vi "設定項目_登録_INI書込サブ.vi"(2 "CSV項目名":T1, 4 "設定クラスタ_設定入力":T5 {"測定モード" items=["単発測定モード", "連続測定モード", "多点測定モード"]}, 5 "セレクション(設定)":string, 6 "エラー入力":errorcluster caption="エラー入力 (エラーなし)", 7 "セレクション(No)":string, 8 "使用ON/OFFボタン_設定入力":T3, 9 "キー(配列No)":string[](array[string]), 10 "No設定クラスタ_設定入力":T4, 11 "Refnum入力":T2 caption="refnum") -> (0 "エラー出力":errorcluster, 3 "Refnum出力":T2 caption="refnum")   [LabVIEW 2021]
uses:
  <vilib>/Utility/config.llb/Config Data RefNum.ctl
  <vilib>/Utility/config.llb/Write Key (Double).vi
  <vilib>/Utility/config.llb/Write Key (String).vi
  <vilib>/Utility/config.llb/Write Key (U32).vi
  <vilib>/Utility/config.llb/Write Key (Boolean).vi
  <vilib>/Utility/config.llb/NI_LVConfig.lvlib
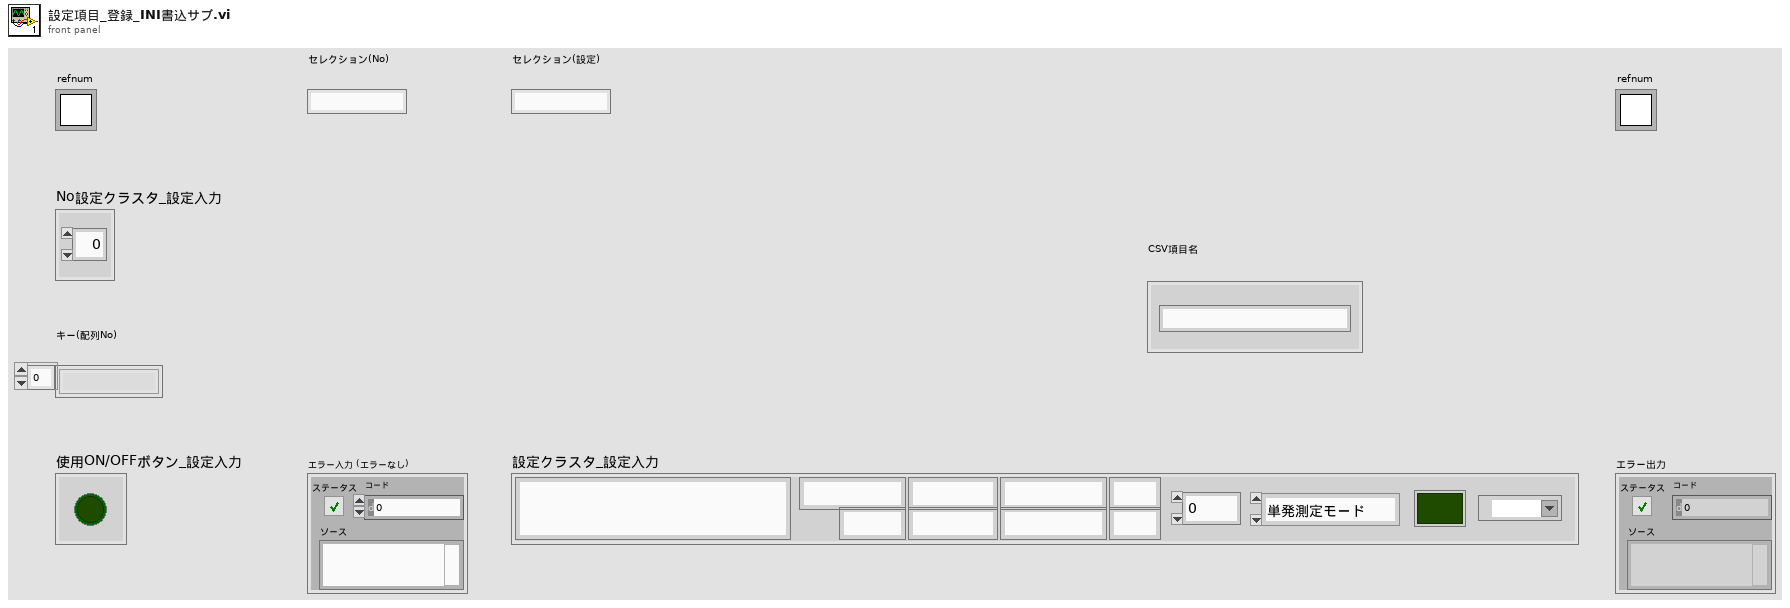
[diagram p1: front panel]
types:
  T1 = typedef "CSV項目名入力.ctl" = cluster{"CSV項目名":string}
  T2 = typedef "NI_LVConfig.lvlib/Config Data RefNum.ctl" = refnum<k1>
  T3 = typedef "ONOFFボタン制御器.ctl" = cluster{"使用ON/OFF":bool}
  T4 = typedef "CH設定表示器.ctl" = cluster{"No. ":dbl}
  T5 = typedef "設定全項目制御器.ctl" = cluster{"規格":string, "規格上限":string, "規格下限":string, "ポートNo.":dbl, "測定モード":u16, "規格単位":string, "品質チェック項目":string, "測定周期":dbl, "実測値MAX":string, "実測値MIN":string, "実測値(MAX)":string, "実測値(MIN)":string, "測定画面表示ボタン":bool, "ゲージポートNo":refnum<visa-resource-name>}
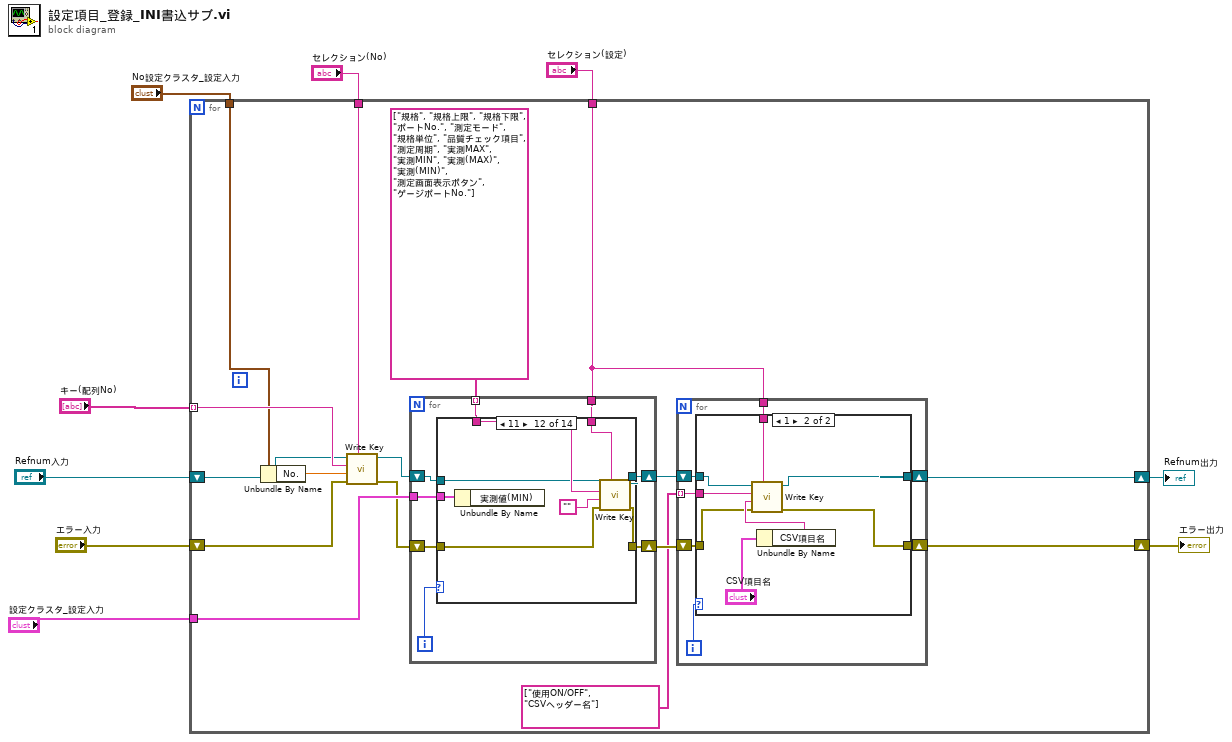
[diagram p0: block diagram]
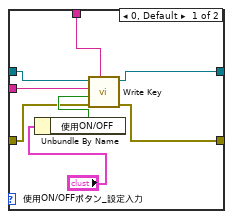
[diagram p2: hidden frame]
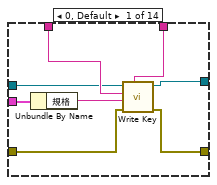
[diagram p3: hidden frame]
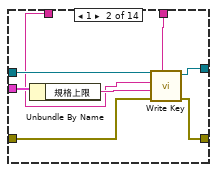
[diagram p4: hidden frame]
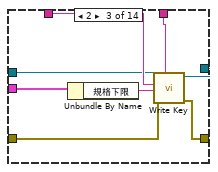
[diagram p5: hidden frame]
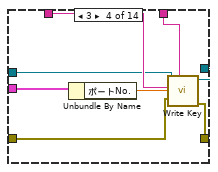
[diagram p6: hidden frame]
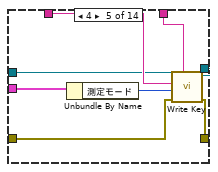
[diagram p7: hidden frame]
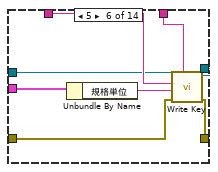
[diagram p8: hidden frame]
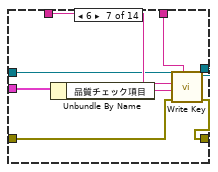
[diagram p9: hidden frame]
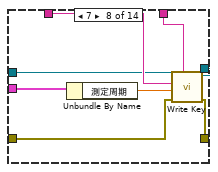
[diagram p10: hidden frame]
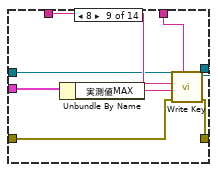
[diagram p11: hidden frame]
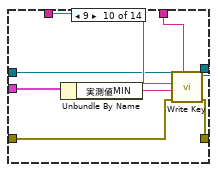
[diagram p12: hidden frame]
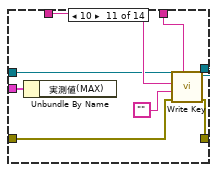
[diagram p13: hidden frame]
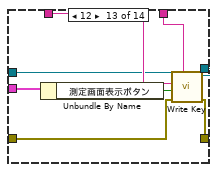
[diagram p14: hidden frame]
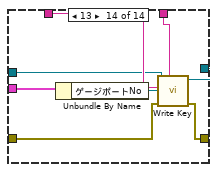
[diagram p15: hidden frame]
diagram:
  n1 = for {
    shift-right: [w23] -> w4
    shift-left: "Refnum入力" -> [w24]
    tunnel: "キー(配列No)" -> [w25] mode=indexing
    shift-right: [w21] -> w5
    shift-left: "エラー入力" -> [w22]
    tunnel: "No設定クラスタ_設定入力" -> [w20]
    tunnel: "設定クラスタ_設定入力" -> [w19]
    tunnel: "セレクション(No)" -> [w18]
    tunnel: "セレクション(設定)" -> [w17]
    n2 = Unbundle By Name(w20) -> ("No."=w16:dbl)
    n3 = call-poly <vilib>:"Write Key.vi"("section"=w18, "error in (no error)"=w22, "value"=w16, "key"=w25, "refnum"=w24) -> ("error out"=w13:errorcluster, "refnum out"=w15:T2)  [unwired: 3 in, 2 out]
    n4 = for {
      shift-right: [w54] -> w14
      shift-left: w15 -> [w56]
      tunnel: string[] ["規格", "規格上限", "規格下限", "ポートNo.", "測定モード", "規格単位", "品質チェック項目", "測定周期", "実測MAX", "実測MIN", "実測(MAX)", "実測(MIN)", "測定画面表示ボタン", "ゲージポートNo."] -> [w55] mode=indexing
      shift-right: [w51] -> w12
      shift-left: w13 -> [w52]
      tunnel: w19 -> [w50]
      tunnel: w17 -> [w49]
      i -> [w53]
      n5 = case shown="11" w53 {
        tunnel: w50 -> [w64 w72 w79 w87 w95 w103 w111 w119 w127 w135 w144 w152 w159 w167]
        tunnel: w55 -> [w62 w69 w78 w86 w94 w102 w110 w118 w126 w134 w143 w151 w158 w166]
        tunnel: w56 -> [w61 w71 w77 w85 w93 w101 w109 w117 w125 w133 w142 w150 w157 w165]
        tunnel: [w60 w67 w76 w84 w92 w100 w108 w116 w124 w132 w141 w149 w156 w164] -> w54
        tunnel: w49 -> [w59 w68 w75 w83 w91 w99 w107 w115 w123 w131 w140 w148 w155 w163]
        tunnel: w52 -> [w58 w66 w74 w82 w90 w98 w106 w114 w122 w130 w139 w147 w154 w162]
        tunnel: [w57 w65 w73 w81 w89 w97 w105 w113 w121 w129 w138 w146 w153 w161] -> w51
        frame 0, Default {
          n6 = Unbundle By Name(w64) -> ("規格"=w63:string)
          n7 = call-poly <vilib>:"Write Key.vi"("section"=w59, "error in (no error)"=w58, "value"=w63, "key"=w62, "refnum"=w61) -> ("error out"=w57:errorcluster, "refnum out"=w60:T2)  [unwired: 1 in, 4 out]
        }
        frame 1 {
          n8 = Unbundle By Name(w72) -> ("規格上限"=w70:string)
          n9 = call-poly <vilib>:"Write Key.vi"("section"=w68, "error in (no error)"=w66, "value"=w70, "key"=w69, "refnum"=w71) -> ("error out"=w65:errorcluster, "refnum out"=w67:T2)  [unwired: 1 in, 4 out]
        }
        frame 2 {
          n10 = Unbundle By Name(w79) -> ("規格下限"=w80:string)
          n11 = call-poly <vilib>:"Write Key.vi"("section"=w75, "error in (no error)"=w74, "value"=w80, "key"=w78, "refnum"=w77) -> ("error out"=w73:errorcluster, "refnum out"=w76:T2)  [unwired: 1 in, 4 out]
        }
        frame 3 {
          n12 = Unbundle By Name(w87) -> ("ポートNo."=w88:dbl)
          n13 = call-poly <vilib>:"Write Key.vi"("section"=w83, "error in (no error)"=w82, "value"=w88, "key"=w86, "refnum"=w85) -> ("error out"=w81:errorcluster, "refnum out"=w84:T2)  [unwired: 3 in, 2 out]
        }
        frame 4 {
          n14 = Unbundle By Name(w95) -> ("測定モード"=w96:u16)
          n15 = call-poly <vilib>:"Write Key.vi"("section"=w91, "error in (no error)"=w90, "value"=w96, "key"=w94, "refnum"=w93) -> ("error out"=w89:errorcluster, "refnum out"=w92:T2)  [unwired: 1 in, 4 out]
        }
        frame 5 {
          n16 = Unbundle By Name(w103) -> ("規格単位"=w104:string)
          n17 = call-poly <vilib>:"Write Key.vi"("section"=w99, "error in (no error)"=w98, "value"=w104, "key"=w102, "refnum"=w101) -> ("error out"=w97:errorcluster, "refnum out"=w100:T2)  [unwired: 1 in, 4 out]
        }
        frame 6 {
          n18 = Unbundle By Name(w111) -> ("品質チェック項目"=w112:string)
          n19 = call-poly <vilib>:"Write Key.vi"("section"=w107, "error in (no error)"=w106, "value"=w112, "key"=w110, "refnum"=w109) -> ("error out"=w105:errorcluster, "refnum out"=w108:T2)  [unwired: 1 in, 4 out]
        }
        frame 7 {
          n20 = Unbundle By Name(w119) -> ("測定周期"=w120:dbl)
          n21 = call-poly <vilib>:"Write Key.vi"("section"=w115, "error in (no error)"=w114, "value"=w120, "key"=w118, "refnum"=w117) -> ("error out"=w113:errorcluster, "refnum out"=w116:T2)  [unwired: 3 in, 2 out]
        }
        frame 8 {
          n22 = Unbundle By Name(w127) -> ("実測値MAX"=w128:string)
          n23 = call-poly <vilib>:"Write Key.vi"("section"=w123, "error in (no error)"=w122, "value"=w128, "key"=w126, "refnum"=w125) -> ("error out"=w121:errorcluster, "refnum out"=w124:T2)  [unwired: 1 in, 4 out]
        }
        frame 9 {
          n24 = Unbundle By Name(w135) -> ("実測値MIN"=w136:string)
          n25 = call-poly <vilib>:"Write Key.vi"("section"=w131, "error in (no error)"=w130, "value"=w136, "key"=w134, "refnum"=w133) -> ("error out"=w129:errorcluster, "refnum out"=w132:T2)  [unwired: 1 in, 4 out]
        }
        frame 10 {
          n26 = Unbundle By Name(w144) -> ()  [unwired: 1 out]
          n27 = call-poly <vilib>:"Write Key.vi"("section"=w140, "error in (no error)"=w139, "value"="", "key"=w143, "refnum"=w142) -> ("error out"=w138:errorcluster, "refnum out"=w141:T2)  [unwired: 1 in, 4 out]
        }
        frame 11 {
          n28 = Unbundle By Name(w152) -> ()  [unwired: 1 out]
          n29 = call-poly <vilib>:"Write Key.vi"("section"=w148, "error in (no error)"=w147, "value"="", "key"=w151, "refnum"=w150) -> ("error out"=w146:errorcluster, "refnum out"=w149:T2)  [unwired: 1 in, 4 out]
        }
        frame 12 {
          n30 = Unbundle By Name(w159) -> ("測定画面表示ボタン"=w160:bool)
          n31 = call-poly <vilib>:"Write Key.vi"("section"=w155, "error in (no error)"=w154, "value"=w160, "key"=w158, "refnum"=w157) -> ("error out"=w153:errorcluster, "refnum out"=w156:T2)  [unwired: 1 in, 4 out]
        }
        frame 13 {
          n32 = Unbundle By Name(w167) -> ("ゲージポートNo"=w168:refnum<visa-resource-name>)
          n33 = call-poly <vilib>:"Write Key.vi"("section"=w163, "error in (no error)"=w162, "value"=w168, "key"=w166, "refnum"=w165) -> ("error out"=w161:errorcluster, "refnum out"=w164:T2)  [unwired: 1 in, 4 out]
        }
      }
    }
    n34 = for {
      shift-right: [w32] -> w23
      shift-left: w14 -> [w29]
      tunnel: string[] ["使用ON/OFF", "CSVヘッダー名"] -> [w30] mode=indexing
      shift-right: [w27] -> w21
      shift-left: w12 -> [w28]
      tunnel: w17 -> [w26]
      i -> [w31]
      n35 = case shown="1" w31 {
        tunnel: [w40 w48] -> w32
        tunnel: w30 -> [w38 w46]
        tunnel: w29 -> [w37 w45]
        tunnel: w26 -> [w36 w44]
        tunnel: w28 -> [w35 w43]
        tunnel: [w34 w42] -> w27
        frame 0, Default {
          n36 = Unbundle By Name("使用ON/OFFボタン_設定入力") -> ("使用ON/OFF"=w39:bool)
          n37 = call-poly <vilib>:"Write Key.vi"("section"=w36, "error in (no error)"=w35, "value"=w39, "key"=w38, "refnum"=w37) -> ("error out"=w34:errorcluster, "refnum out"=w40:T2)  [unwired: 1 in, 4 out]
        }
        frame 1 {
          n38 = Unbundle By Name("CSV項目名") -> ("CSV項目名"=w47:string)
          n39 = call-poly <vilib>:"Write Key.vi"("section"=w44, "error in (no error)"=w43, "value"=w47, "key"=w46, "refnum"=w45) -> ("error out"=w42:errorcluster, "refnum out"=w48:T2)  [unwired: 1 in, 4 out]
        }
      }
    }
  }
  "エラー出力" <- w5
  "Refnum出力" <- w4
